vi "Bundle Script_In Place Rearrange.vi"(10 "Displayed Items":string[](array[string]), 11 "Affected Items":T1) -> (0 "error out":errorcluster)   [LabVIEW 2023]
doc: "Tag tree tags as nput, as these contain the original indices, which are used for reordering the wires and labels of the bundle or unbundle by name structures"
uses:
  top/BundleMagic.ctl
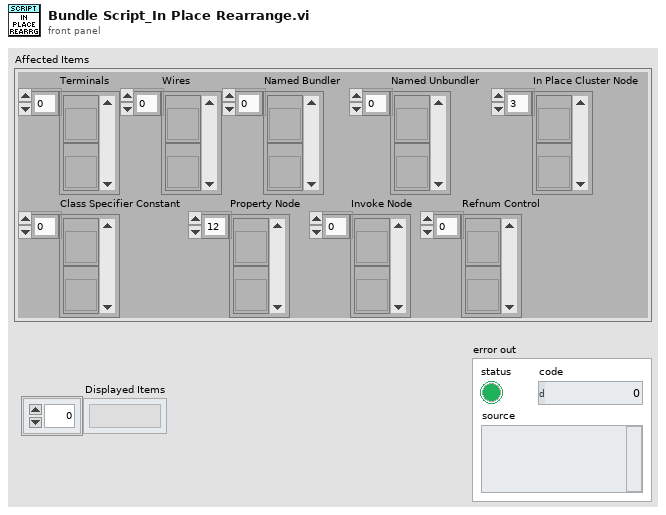
[diagram p1: front panel]
types:
  T1 = typedef "BundleMagic.ctl" = cluster{"Terminals":refnum<vi>[], "Wires":refnum<vi>[], "Named Bundler":refnum<vi>[], "Named Unbundler":refnum<vi>[], "In Place Cluster Node":refnum<vi>[], "Class Specifier Constant":refnum<vi>[], "Property Node":refnum<vi>[], "Invoke Node":refnum<vi>[], "Refnum Control":refnum<vi>[]}
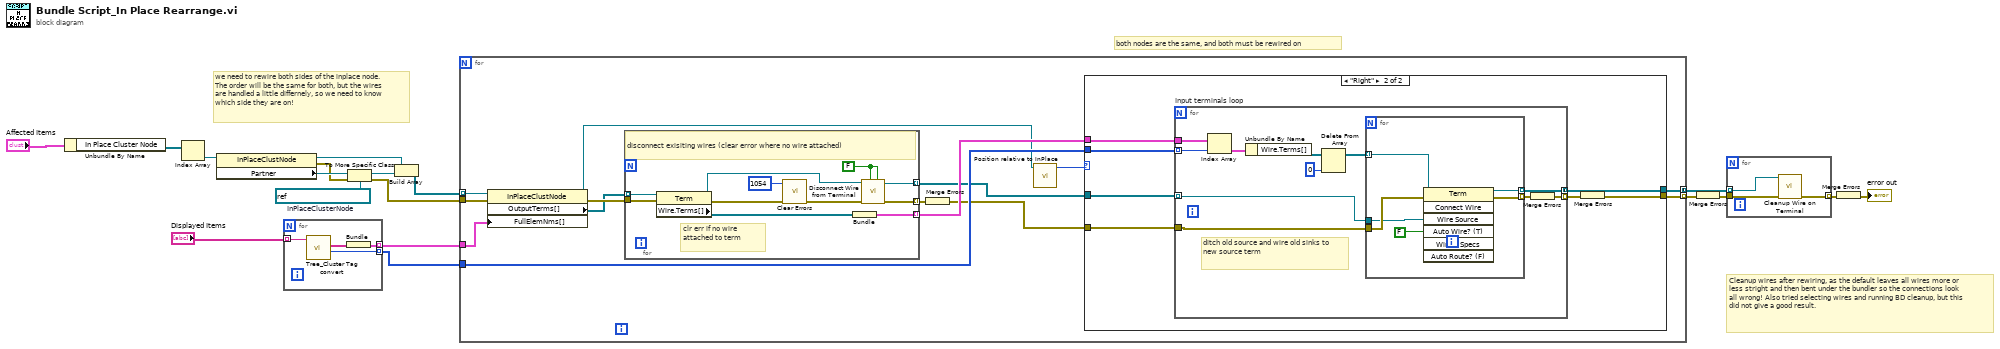
[diagram p0: block diagram]
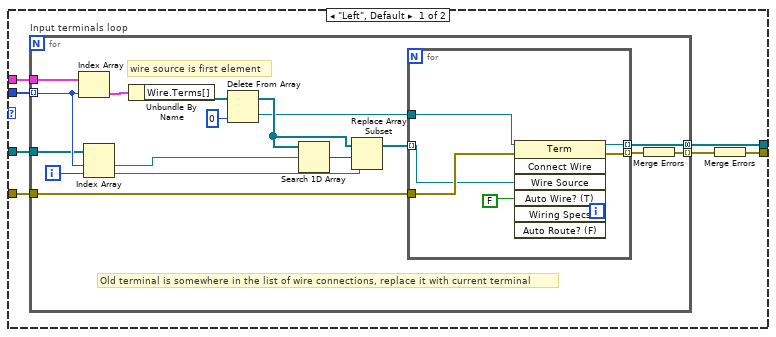
[diagram p2: hidden frame]
diagram:
  w13 = refnum<vi> refnum  # InPlaceClusterNode
  # "we need to rewire both sides of the inplace node. The order will be the same for both, but the wires are handled a little differnely, so we need to know which side they are on!"
  # "both nodes are the same, and both must be rewired on"
  # "Cleanup wires after rewiring, as the default leaves all wires more or less stright and then bent under the bundler so the connections look all wrong! Also tried selecting wires and running BD cleanup, but this did not give a good result."
  n1 = Unbundle By Name("Affected Items") -> ("In Place Cluster Node"=w16:refnum<vi>[])
  n2 = Index Array(array=w16) -> (element=w14:refnum<vi>)  [unwired: 1 in]
  n3 = property class="InPlaceClustNode"(reference=w14) -> (reference out=w11:refnum<vi>, error out=w2:errorcluster, "Partner"=w12:refnum<vi>)  [unwired: 1 in]
  n4 = for {
    tunnel: "Displayed Items" -> [w22] mode=indexing
    tunnel: [w19] -> w8 mode=indexing
    tunnel: [w20] -> w18 mode=indexing
    n5 = call "Tree_Cluster Tag convert.vi"("Tag"=w22) -> ("Index"=w20:u32, "Tree Nest"=w21:string[])  [unwired: 5 in, 4 out]
    n6 = Bundle("Tree Nest"=w21) -> (w19:cluster{"Tree Nest":string[]})  [unwired: 1 in]
  }
  n7 = To More Specific Class(target class=w13, reference=w12, error in=w2) -> (specific class reference=w10:refnum<vi>, error out=w1:errorcluster)
  n8 = Build Array(w11, w10) -> (w9:refnum<vi>[])
  n9 = for {
    tunnel: w18 -> [w35]
    tunnel: w9 -> [w34] mode=indexing
    tunnel: w8 -> [w33]
    tunnel: [w26] -> w6 mode=concatenating
    tunnel: [w25] -> w5 mode=indexing
    tunnel: w1 -> [w23]
    n10 = property class="InPlaceClustNode"(reference=w34, error in=w23, "FullElemNms[]"=w33) -> (reference out=w27:refnum<vi>, error out=w31:errorcluster, "OutputTerms[]"=w29:refnum<vi>[])
    n11 = for {
      tunnel: w29 -> [w47] mode=indexing
      tunnel: [w45] -> w36 mode=indexing
      tunnel: [w41] -> w30 mode=indexing
      tunnel: w31 -> [w44]
      tunnel: [w40] -> w28 mode=indexing
      w39 = FALSE ("Clean Up wire")
      # "clr err if no wire attached to term"
      # "disconnect exisiting wires (clear error where no wire attached)"
      n12 = property class="Term"(reference=w47, error in=w44) -> (reference out=w42:refnum<vi>, error out=w43:errorcluster, "Wire.Terms[]"=w46:refnum<vi>[])
      n13 = call <vilib>:"Clear Errors.vi"("error in (no error)"=w43, "specific error code to clear (0: all)"=1054) -> ("error out"=w38:errorcluster)  [unwired: 4 in, 1 out]
      n14 = Bundle("Wire.Terms[]"=w46) -> (w45:cluster{"Wire.Terms[]":refnum<vi>[]})  [unwired: 1 in]
      n15 = call "Disconnect Wire from Terminal.vi"("Remove Loose Ends"=w39, "Clean Up wire"=w39, "error in"=w38, "Terminal in"=w42) -> ("error out"=w41:errorcluster, "Terminal out"=w40:refnum<vi>)  [unwired: 3 in, 3 out]
    }
    n16 = Merge Errors(w30) -> (w24:errorcluster)
    n17 = call "Position relative to InPlace.vi"("InPlaceClusterNode in"=w27) -> ("Position"=w32:enum16{"Left", "Top", "Right", "Bottom"})  [unwired: 10 in]
    n18 = case shown="\"Right\"" w32 {
      tunnel: w36 -> [w54 w84]
      tunnel: w35 -> [w53 w83]
      tunnel: [w52 w82] -> w26
      tunnel: w24 -> [w51 w81]
      tunnel: w28 -> [w50 w80]
      tunnel: [w48 w78] -> w25
      frame "Left", Default {
        n19 = for "Input terminals loop" {
          tunnel: w54 -> [w63]
          tunnel: w53 -> [w62] mode=indexing
          tunnel: w50 -> [w58]
          tunnel: w51 -> [w71]
          tunnel: [w70] -> w52 mode=concatenating
          tunnel: [w55] -> w49 mode=indexing
          i -> [w59]
          # "wire source is first element"
          # "Old terminal is somewhere in the list of wire connections, replace it with current terminal"
          n20 = Index Array(array=w63, index=w62) -> (element=w68:cluster{"Wire.Terms[]":refnum<vi>[]})
          n21 = Index Array(array=w58, index #1=w62, index #2=w59) -> (element #1=w57:refnum<vi>, element #2=w56:refnum<vi>)
          n22 = Unbundle By Name(w68) -> ("Wire.Terms[]"=w67:refnum<vi>[])
          n23 = Delete From Array(array=w67, index=0) -> (deleted portion=w61:refnum<vi>, array with subset deleted=w65:refnum<vi>[])  [unwired: 1 in]
          n24 = Search 1D Array(1D array=w65, element=w57) -> (index of element=w66:i32)  [unwired: 1 in]
          n25 = Replace Array Subset(array=w65, new element=w56, index=w66) -> (w60:refnum<vi>[])
          n26 = for {
            tunnel: w71 -> [w77]
            tunnel: [w73] -> w70 mode=indexing
            tunnel: [w72] -> w69 mode=indexing
            tunnel: w61 -> [w75]
            tunnel: w60 -> [w74] mode=indexing
            n27 = invoke class="Term" method="Connect Wire"(reference=w75, error in=w77, "Wire Source"=w74, "Auto Wire? (T)"=FALSE) -> (reference out=w73:refnum<vi>, error out=w72:errorcluster)  [unwired: 3 in, 5 out]
          }
          n28 = Merge Errors(w69) -> (w55:errorcluster)
        }
        n29 = Merge Errors(w49) -> (w48:errorcluster)
      }
      frame "Right" {
        n30 = for "Input terminals loop" {
          tunnel: w84 -> [w94]
          tunnel: w83 -> [w92] mode=indexing
          tunnel: w80 -> [w87] mode=indexing
          tunnel: w81 -> [w95]
          tunnel: [w89] -> w82 mode=concatenating
          tunnel: [w85] -> w79 mode=indexing
          # "ditch old source and wire old sinks to new source term"
          n31 = Index Array(array=w94, index=w92) -> (element=w93:cluster{"Wire.Terms[]":refnum<vi>[]})
          n32 = Unbundle By Name(w93) -> ("Wire.Terms[]"=w91:refnum<vi>[])
          n33 = Delete From Array(array=w91, index=0) -> (array with subset deleted=w86:refnum<vi>[])  [unwired: 1 in, 1 out]
          n34 = for {
            tunnel: w95 -> [w101]
            tunnel: [w97] -> w89 mode=indexing
            tunnel: [w96] -> w88 mode=indexing
            tunnel: w87 -> [w99]
            tunnel: w86 -> [w98] mode=indexing
            n35 = invoke class="Term" method="Connect Wire"(reference=w98, error in=w101, "Wire Source"=w99, "Auto Wire? (T)"=FALSE) -> (reference out=w97:refnum<vi>, error out=w96:errorcluster)  [unwired: 3 in, 5 out]
          }
          n36 = Merge Errors(w88) -> (w85:errorcluster)
        }
        n37 = Merge Errors(w79) -> (w78:errorcluster)
      }
    }
  }
  n38 = Merge Errors(w5) -> (w3:errorcluster)
  n39 = for {
    tunnel: w6 -> [w102] mode=indexing
    tunnel: w3 -> [w104]
    tunnel: [w103] -> w7 mode=indexing
    n40 = call "Cleanup Wire on Terminal.vi"("error in"=w104, "Terminal in"=w102) -> ("error out"=w103:errorcluster)  [unwired: 7 in, 2 out]
  }
  n41 = Merge Errors(w7) -> (→"error out":errorcluster)
